vi "Convert Temperatures.vi"() -> ()   [LabVIEW 2012]
panel:
  out "温度（绝对温度）":dbl[](array[numeric])
  in  "温度（摄氏度）":dbl[](array[numeric])=[-120.0, -200.0, -75.0, -45.0]
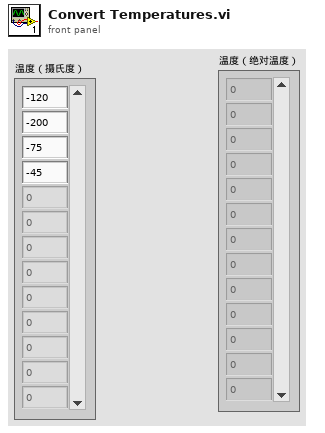
[diagram p1: front panel]
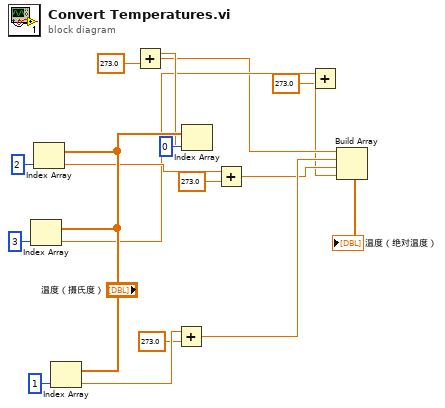
[diagram p0: block diagram]
diagram:
  n1 = Index Array ("索引数组")(array="温度（摄氏度）", index=3 ("索引")) -> (element=w10:dbl)
  n2 = Index Array ("索引数组")(array="温度（摄氏度）", index=2 ("索引")) -> (element=w11:dbl)
  n3 = Index Array ("索引数组")(array="温度（摄氏度）", index=1 ("索引")) -> (element=w12:dbl)
  n4 = Add ("加")(x=w12, y=273.0) -> (x+y=w8:dbl)
  n5 = Index Array ("索引数组")(array="温度（摄氏度）", index=0 ("索引")) -> (element=w13:dbl)
  n6 = Add ("加")(x=w13, y=273.0) -> (x+y=w9:dbl)
  n7 = Add ("加")(x=w11, y=273.0) -> (x+y=w7:dbl)
  n8 = Add ("加")(x=w10, y=273.0) -> (x+y=w6:dbl)
  n9 = Build Array ("创建数组")(w9, w8, w7, w6) -> (→"温度（绝对温度）":dbl[])
